vi "Copy Scripting API to Installed Location.vi"(5 "Files Generated by Build":path[](array[path]), 6 "Top Level/Always Included VIs":path[](array[path]), 7 "Destination Path":path, 8 "error in (no error)":errorcluster, 9 "Target Name":string, 10 "Build Specification Name":string, 11 "Project Path":path) -> (0 "error out":errorcluster)   [LabVIEW 2017]
doc: "This VI is called after each run of a build specification. The VI will copy the generated LLB (Engine or System Explorer) into the VeriStand Custom Device folder (...\\Documents\\National Instruments\\NI VeriStand 2013...)."
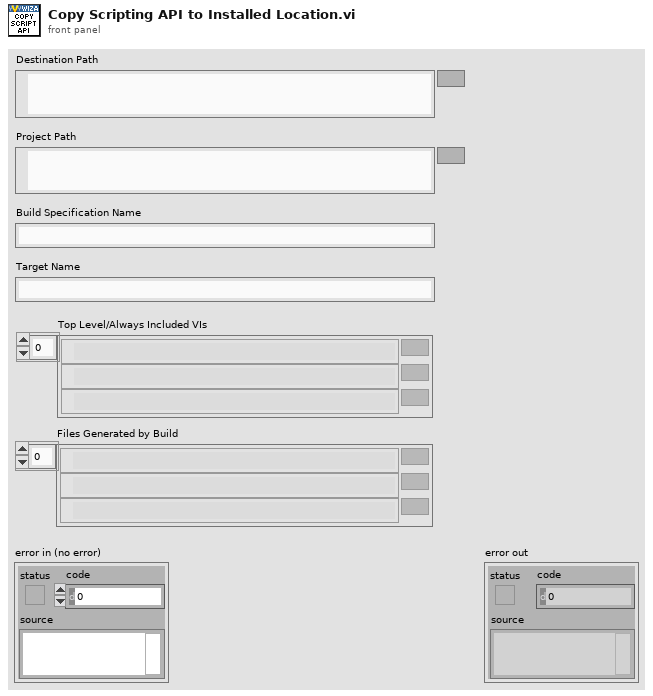
[diagram p1: front panel]
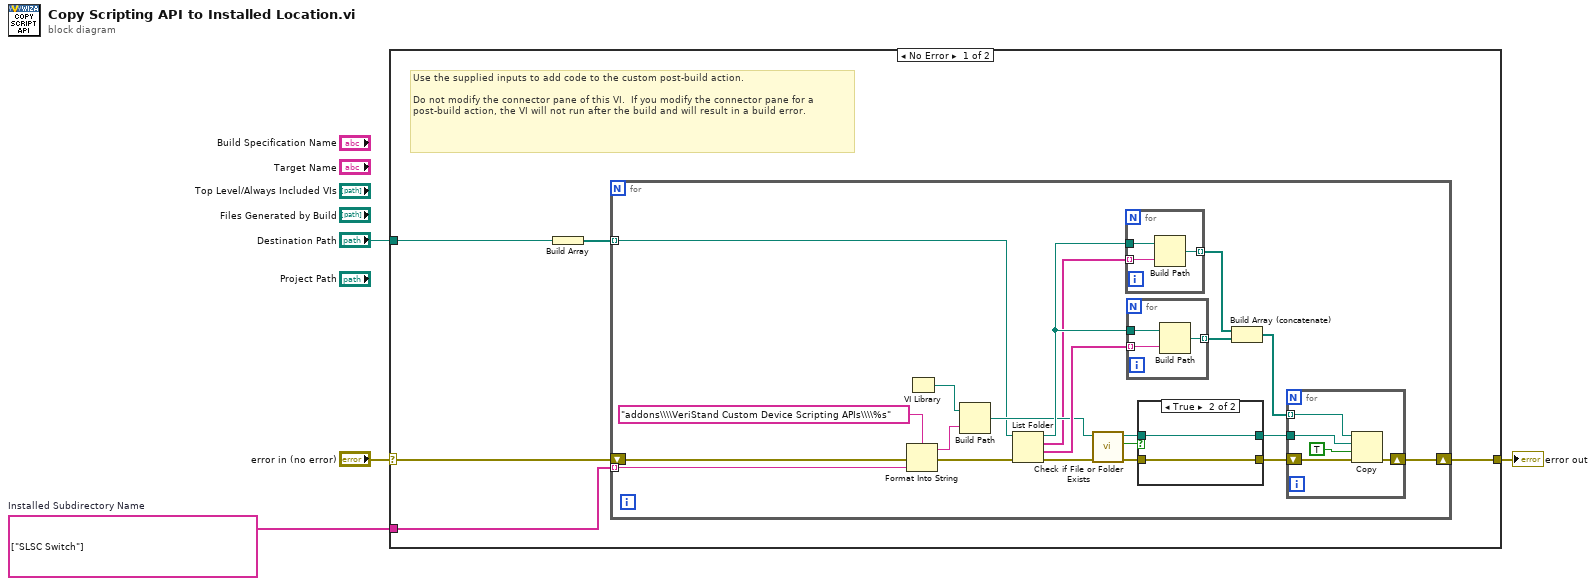
[diagram p0: block diagram]
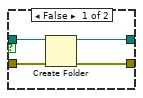
[diagram p2: hidden frame]
diagram:
  w3 = string[] ["SLSC Switch"]  # Installed Subdirectory Name
  n1 = case shown="No Error" "error in (no error)" {
    selector: "error in (no error)" -> [w9 w48]
    tunnel: [w7 w48] -> w2
    tunnel: w3 -> [w8 _]
    tunnel: "Destination Path" -> [w5 _]
    frame No Error {
      # "Use the supplied inputs to add code to the custom post-build action.\n\nDo not modify the connector pane of this VI.  If you modify the connector pane for a post-build action, the VI will not run after the build and will result in a build error."
      n2 = Build Array(w5) -> (w6:path[])
      n3 = for {
        tunnel: w8 -> [w16] mode=indexing
        tunnel: w6 -> [w10] mode=indexing
        shift-right: [w11] -> w7
        shift-left: w9 -> [w18]
        n4 = Format Into String(format string="addons\\\\VeriStand Custom Device Scripting APIs\\\\%s" ("name or relative path"), error in=w18, w16) -> (resulting string=w21:string, error out=w17:errorcluster)  [unwired: 1 in]
        n5 = VI Library() -> (path=w12:path)
        n6 = Build Path(base path=w12, name or relative path=w21) -> (appended path=w19:path)
        n7 = List Folder(path=w10, error in=w17) -> (path out=w24:path, filenames=w14:string[], folder names=w25:string[], error out=w22:errorcluster)  [unwired: 2 in]
        n8 = call <vilib>:"Check if File or Folder Exists.vi"("error in (no error)"=w22, "path"=w19) -> ("error out"=w26:errorcluster, "file or folder exists?"=w28:bool, "dup path"=w27:path)  [unwired: 7 in]
        n9 = for {
          tunnel: w14 -> [w46] mode=indexing
          tunnel: w24 -> [w47]
          tunnel: [w45] -> w30 mode=indexing
          n10 = Build Path(base path=w47, name or relative path=w46) -> (appended path=w45:path)
        }
        n11 = for {
          tunnel: w25 -> [w43] mode=indexing
          tunnel: w24 -> [w44]
          tunnel: [w42] -> w23 mode=indexing
          n12 = Build Path(base path=w44, name or relative path=w43) -> (appended path=w42:path)
        }
        n13 = case shown="True" w28 {
          tunnel: w27 -> [w34 w36]
          tunnel: w26 -> [w33 w35]
          tunnel: [w32 w36] -> w13
          tunnel: [w31 w35] -> w15
          frame False {
            n14 = Create Folder(path (use dialog)=w34, error in=w33) -> (created path=w32:path, error out=w31:errorcluster)  [unwired: 1 in, 1 out]
          }
          frame True {
          }
        }
        n15 = Build Array (concatenate)(w30, w23) -> (w29:path[])
        n16 = for {
          tunnel: w29 -> [w38] mode=indexing
          shift-right: [w39] -> w11
          shift-left: w15 -> [w40]
          tunnel: w13 -> [w37]
          n17 = Copy(8:w40, 9:TRUE ("overwrite (F)"), 10:w37, 11:w38) -> (0:w39:errorcluster)  [unwired: 1 in, 2 out]
        }
      }
    }
    frame Error {
    }
  }
  "error out" <- w2
